vi "Power_spectrum_Autocorrelation.vi"(5 "Spectrum input array":dbl[](array[numeric]) format="%.2f", 7 "Time Trace":T2, 8 "Cluster in":T3={"Colour"=0, "Inst type"=enum."Pitot-static tube", "Inst name"="Manometer voltage", "Symbol"="U", "Code name"="", "Extra Info"="U", "Inst Array"=enum."PWA", "Extra Titles"=[], "Extra Values"=[], "U"=0.0, "u^2"=0.0, "u^3"=0.0, "u^4"=0.0, "Skew_u"=0.0, "Kurt_u"=0.0, "Sd Error in Mean"=0.0, "% u'/U"=0.0, "X"=0.0, "Y"=0.0, "Z"=0.0, "Timescale integral Estimate"=0.0, "Sd Error in Variance"=0.0, "Calib File"=path "", "Calib Constants"=[], "Output Position"=FALSE, "Full Stats"=FALSE, "Av Sampling Rate"=0.0, "Av No of Samples"=0.0, "Total Meas Time (s)"=0.0, "ADAM Ch Name"="", "Max value"=0.0, "Min value"=0.0} {"Sd Error in Variance" format="%.2f"; "Skew_u" format="%.2f"; "% u'/U" format="%.2f"; "Sd Error in Mean" format="%.2f"; "Kurt_u" format="%.2f"; "u^4" format="%.2f"; "u^3" format="%.2f"; "U" format="%.2f"; "u^2" format="%.2f"}) -> (0 "Spectrum output array":dbl[](array[numeric]) format="%.2f", 1 "Autocorrelation":T1, 2 "Spectra":T1, 3 "Cluster Out":T3={"Colour"=0, "Inst type"=enum."Pitot-static tube", "Inst name"="Manometer voltage", "Symbol"="U", "Code name"="", "Extra Info"="U", "Inst Array"=enum."PWA", "Extra Titles"=[], "Extra Values"=[], "U"=0.0, "u^2"=0.0, "u^3"=0.0, "u^4"=0.0, "Skew_u"=0.0, "Kurt_u"=0.0, "Sd Error in Mean"=0.0, "% u'/U"=0.0, "X"=0.0, "Y"=0.0, "Z"=0.0, "Timescale integral Estimate"=0.0, "Sd Error in Variance"=0.0, "Calib File"=path "", "Calib Constants"=[], "Output Position"=FALSE, "Full Stats"=FALSE, "Av Sampling Rate"=0.0, "Av No of Samples"=0.0, "Total Meas Time (s)"=0.0, "ADAM Ch Name"="", "Max value"=0.0, "Min value"=0.0} {"Sd Error in Variance" format="%.2f"; "Skew_u" format="%.2f"; "% u'/U" format="%.2f"; "Sd Error in Mean" format="%.2f"; "Kurt_u" format="%.2f"; "u^4" format="%.2f"; "u^3" format="%.2f"; "U" format="%.2f"; "u^2" format="%.2f"})   [LabVIEW 2016]
uses:
  Controls/Analysis_info_cluster.ctl
  Controls/Inst_type.ctl
  Controls/Instrument_Array.ctl
  Controls/Time_Trace_Cluster.ctl
  Controls/XY_Plot_Cluster.ctl
  Globals/Meas_global.vi
  <vilib>/gmath/NI_Gmath.lvlib
panel:
  out "Numeric":dbl
  out "size(s)":i32
  out "XY Graph 2":cluster{dbl[], dbl[]}(graph)
  in  "method":i32(ring) items=["nearest", "linear", "spline", "cubic Hermite", "Lagrange"]
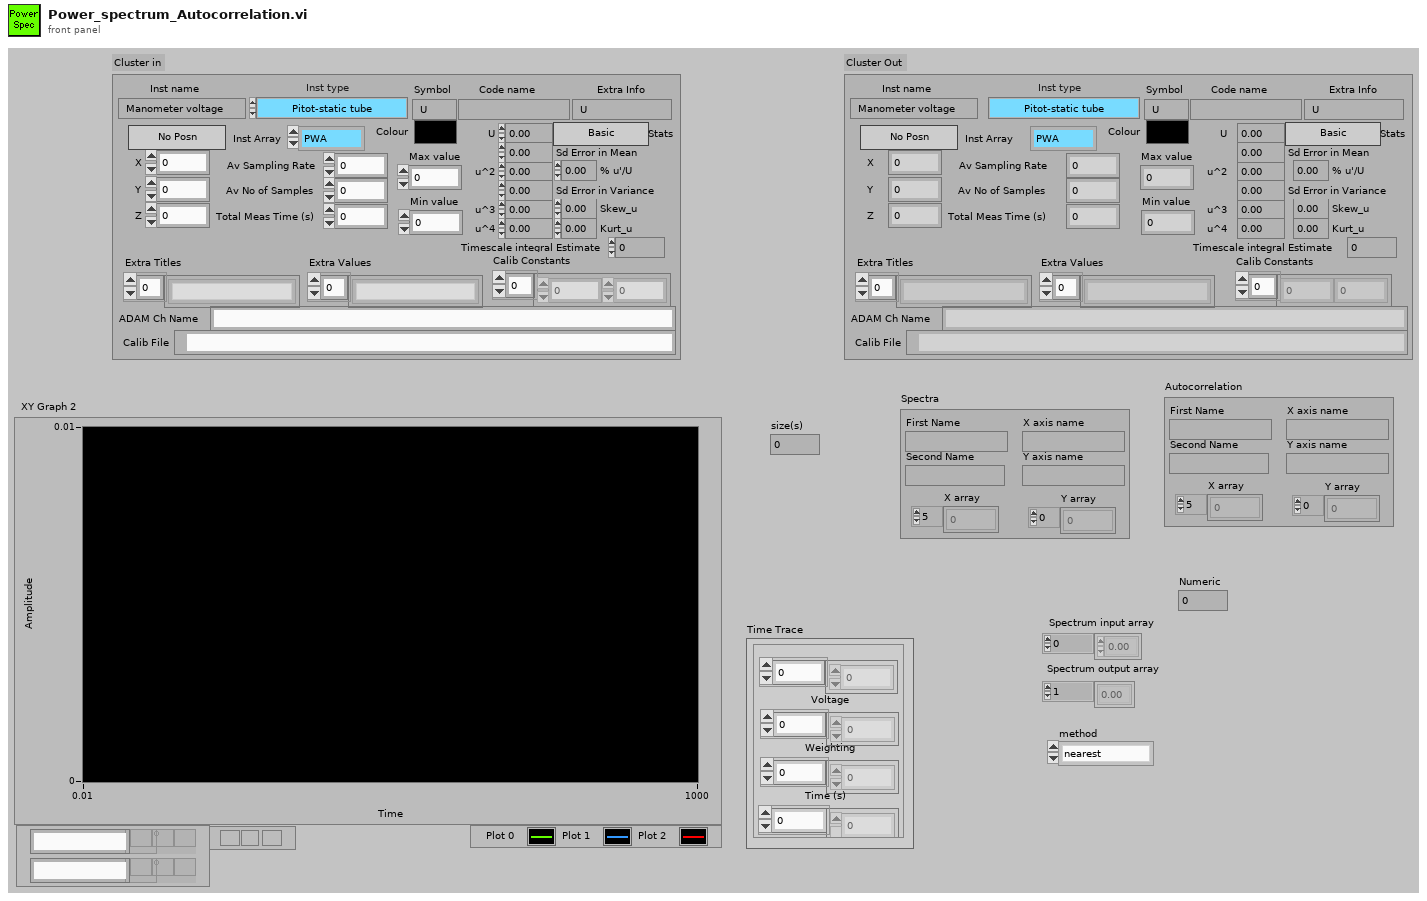
[diagram p1: front panel]
types:
  T1 = typedef "XY_Plot_Cluster.ctl" = cluster{"First Name":string, "Second Name":string, "X axis name":string, "Y axis name":string, "X array":dbl[], "Y array":dbl[]}
  T2 = typedef "Time_Trace_Cluster.ctl" = cluster{"Weighting":dbl[], "Time (s)":dbl[], "Voltage":dbl[], "Eng Values":dbl[]}
  T3 = typedef "Analysis_info_cluster.ctl" = cluster{"Colour":u32, "Inst type":T4, "Inst name":string, "Symbol":string, "Code name":string, "Extra Info":string, "Inst Array":T5, "Extra Titles":string[], "Extra Values":string[], "U":dbl, "u^2":dbl, "u^3":dbl, "u^4":dbl, "Skew_u":dbl, "Kurt_u":dbl, "Sd Error in Mean":dbl, "% u'/U":dbl, "X":dbl, "Y":dbl, "Z":dbl, "Timescale integral Estimate":dbl, "Sd Error in Variance":dbl, "Calib File":path, "Calib Constants":dbl[], "Output Position":bool, "Full Stats":bool, "Av Sampling Rate":dbl, "Av No of Samples":dbl, "Total Meas Time (s)":dbl, "ADAM Ch Name":string, "Max value":dbl, "Min value":dbl}
  T4 = typedef "Inst_type.ctl" = enum16{"Propeller anemometer", "Raw voltage", "Pressure Transducer", "Pitot-static tube", "Preston tube", "Hot wire", "Cross wire 1", "Cross wire 2", "Generic Linear", "Generic Polynomial", "Generic BackPoly", "Fast FID", "Thermocouple", "Cold wire", "Pulsed Wire", "LDA Vel", "LDA Tran time", "LDA Arr time", "Microphone"}
  T5 = typedef "Instrument_Array.ctl" = enum16{"PWA", "LDA", "Analogue"}
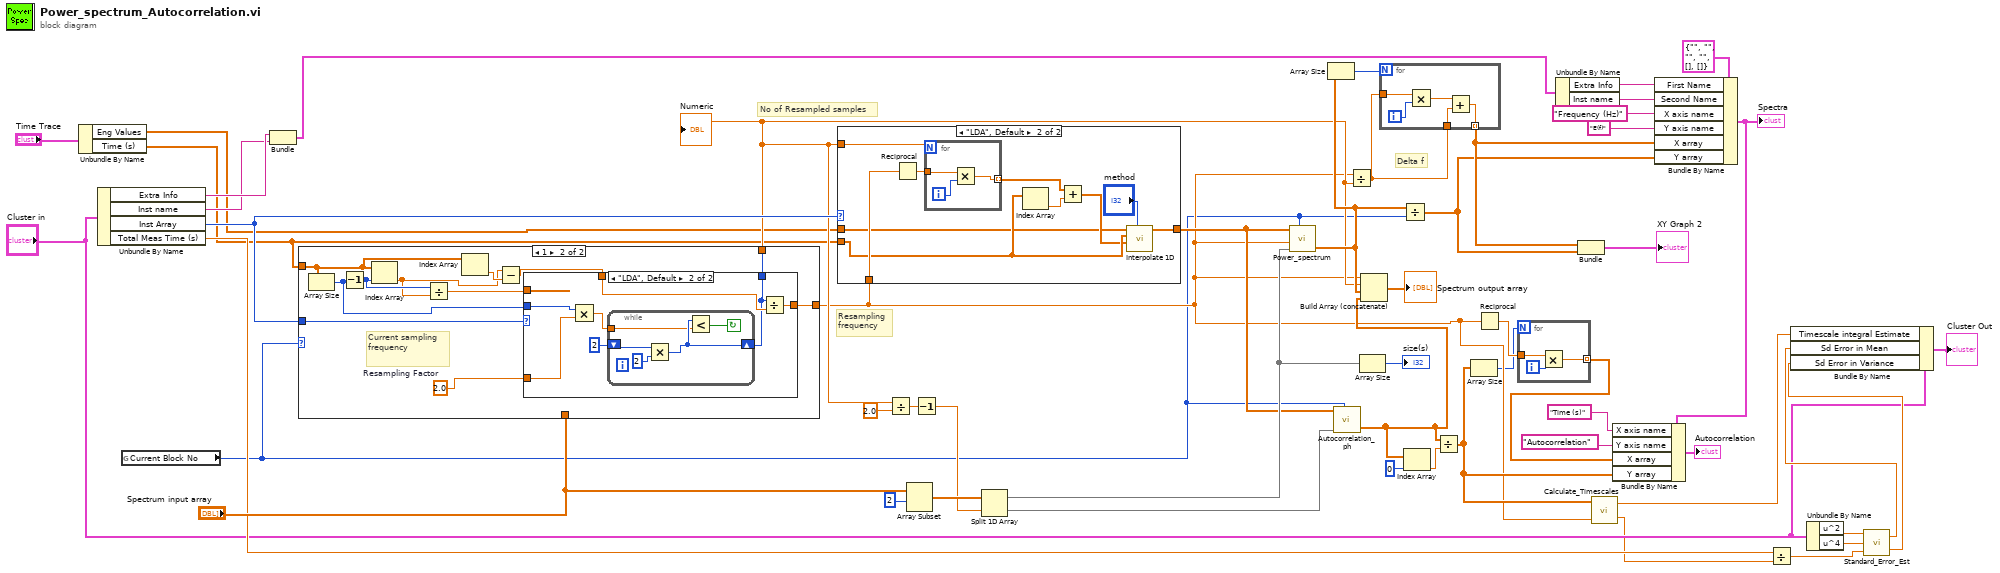
[diagram p0: block diagram]
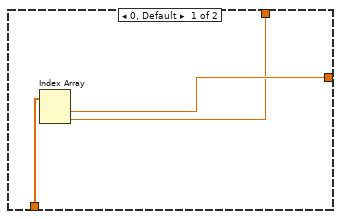
[diagram p2: hidden frame]
diagram:
  # "No of Resampled samples"
  # "Resampling\nfrequency"
  # "Delta f"
  n1 = Unbundle By Name("Time Trace") -> ("Eng Values"=w9:dbl[], "Time (s)"=w5:dbl[])
  n2 = Unbundle By Name("Cluster in") -> ("Extra Info"=w47:string, "Inst name"=w45:string, "Inst Array"=w51:T5, "Total Meas Time (s)"=w11:dbl)
  n3 = global read "Meas_global.vi" "Current Block No"() -> (w3:i32)
  n4 = Bundle("Extra Info"=w47, "Inst name"=w45) -> (w46:cluster{"Extra Info":string, "Inst name":string})  [unwired: 1 in]
  n5 = case shown="1" w3 {
    tunnel: w5 -> [_ w60]
    tunnel: [w55 w65] -> w18
    tunnel: "Spectrum input array" -> [w56 _]
    tunnel: w51 -> [_ w66]
    tunnel: [w54 w63] -> w34
    frame 0, Default {
      n6 = Index Array(array=w56) -> (element #1=w55:dbl, element #2=w54:dbl)  [unwired: 2 in]
    }
    frame 1 {
      w61 = 2.0  # Resampling Factor
      # "Current sampling\nfrequency"
      n7 = Array Size(array=w60) -> (size(s)=w62:i32)
      n8 = Decrement(x=w62) -> (x-1=w64:i32)
      n9 = Index Array(array=w60, index=w64) -> (element=w57:dbl)
      n10 = Divide(x=w64, y=w57) -> (x/y=w67:dbl)
      n11 = Index Array(array=w60) -> (element=w59:dbl)  [unwired: 1 in]
      n12 = Subtract(x=w57, y=w59) -> (x-y=w58:dbl)
      n13 = case shown="\"LDA\", Default" w66 {
        tunnel: w67 -> [w69 _]
        tunnel: w58 -> [_ w76]
        tunnel: [w69 w75] -> w65
        tunnel: w62 -> [w68 w73]
        tunnel: [w68 w72] -> w63
        tunnel: w61 -> [_ w71]
        frame "Analogue" {
        }
        frame "LDA", Default {
          n14 = Multiply(x=w73, y=w71) -> (x*y=w74:dbl)
          n15 = while {
            shift-right: [w79] -> w72
            shift-left: 2 -> [w81]
            tunnel: w74 -> [w77]
            stop <- w78 continue-if-true
            n16 = Multiply(x=w81, y=2) -> (x*y=w79:i32)
            n17 = Less?(x=w79, y=w77) -> (x < y?=w78:bool)
          }
          n18 = Divide(x=w72, y=w76) -> (x/y=w75:dbl)
        }
      }
    }
  }
  "Numeric" <- w34
  n19 = case shown="\"LDA\", Default" w51 {
    tunnel: w9 -> [w82 w83]
    tunnel: w5 -> [_ w87]
    tunnel: [w82 w91] -> w29
    tunnel: w34 -> [_ w90]
    tunnel: w18 -> [_ w88]
    frame "Analogue" {
    }
    frame "LDA", Default {
      n20 = Reciprocal(x=w88) -> (1/x=w89:dbl)
      n21 = for {
        N: w90 -> [_]
        tunnel: w89 -> [w95]
        tunnel: [w93] -> w85 mode=indexing
        i -> [w94]
        n22 = Multiply(x=w95, y=w94) -> (x*y=w93:dbl)
      }
      n23 = Index Array(array=w87) -> (element=w86:dbl)  [unwired: 1 in]
      n24 = Add(x=w85, y=w86) -> (x+y=w84:dbl[])
      n25 = call <vilib>:"Interpolate 1D.vi"("method"="method", "xi"=w84, "X"=w87, "Y"=w83) -> ("yi"=w91:dbl[])  [unwired: 2 in, 5 out]
    }
  }
  n26 = Divide(x=w34, y=2.0) -> (x/y=w32:dbl)
  n27 = Array Subset(array="Spectrum input array", index=2) -> (w35:dbl[])  [unwired: 1 in]
  n28 = Decrement(x=w32) -> (x-1=w31:dbl)
  n29 = Split 1D Array(array=w35, index=w31) -> (first subarray=w30:dbl[], second subarray=w28:dbl[])
  n30 = call "Power_spectrum.vi"("U"=w29, "Sampling frequency"=w18, "Spectrum input array"=w30, "Block No"=w3) -> ("Spectrum Accumulator array"=w39:dbl[])  [unwired: 1 in, 2 out]
  n31 = Array Size(array=w39) -> (size(s)=w49:i32)
  n32 = call "Autocorrelation_ph.vi"("X"=w29, "Autocorrelation of X"=w28, "Block No"=w3) -> ("Autocorrelation of X"=w25:dbl[])  [unwired: 2 in, 1 out]
  n33 = Divide(x=w18, y=w34) -> (x/y=w50:dbl)
  n34 = Array Size(array=w30) -> (size(s)=→"size(s)":i32)
  n35 = Build Array (concatenate)(w18, w34, w39, w25) -> (→"Spectrum output array":dbl[])
  n36 = for {
    N: w49 -> [_]
    tunnel: w50 -> [w100]
    tunnel: w50 -> [w97]
    tunnel: [w96] -> w40 mode=indexing
    i -> [w99]
    n37 = Multiply(x=w100, y=w99) -> (x*y=w98:dbl)
    n38 = Add(x=w98, y=w97) -> (x+y=w96:dbl)
  }
  n39 = Divide(x=w39, y=w3) -> (x/y=w38:dbl[])
  n40 = Index Array(array=w25, index=0 ("Index")) -> (element=w26:dbl)
  n41 = Divide(x=w25, y=w26) -> (x/y=w20:dbl[])
  n42 = Array Size(array=w20) -> (size(s)=w17:i32)
  n43 = Reciprocal(x=w18) -> (1/x=w22:dbl)
  n44 = for {
    N: w17 -> [_]
    tunnel: w22 -> [w102]
    tunnel: [w101] -> w21 mode=indexing
    i -> [w103]
    n45 = Multiply(x=w102, y=w103) -> (x*y=w101:dbl)
  }
  n46 = Unbundle By Name(w46) -> ("Extra Info"=w44:string, "Inst name"=w43:string)
  n47 = Bundle(w40, w38) -> (→"XY Graph 2":cluster{dbl[], dbl[]})  [unwired: 1 in]
  n48 = call "Calculate_Timescales.vi"("Sampling Frequency (Hz)"=w18, "Autocorrelation"=w20) -> ("Time between Independant samples"=w1:dbl, "Timescale estimate (s)"=w2:dbl)  [unwired: 1 in]
  n49 = Bundle By Name(cluster=T1 {"First Name"="", "Second Name"="", "X axis name"="", "Y axis name"="", "X array"=[], "Y array"=[]} ("element"), "First Name"=w44, "Second Name"=w43, "X axis name"="Frequency (Hz)", "Y axis name"="E(f)", "X array"=w40, "Y array"=w38) -> (w7:T1)
  "Spectra" <- w7
  n50 = Bundle By Name(cluster=w7, "X axis name"="Time (s)", "Y axis name"="Autocorrelation", "X array"=w21, "Y array"=w20) -> (→"Autocorrelation":T1)
  n51 = Divide(x=w11, y=w1) -> (x/y=w14:dbl)
  n52 = Unbundle By Name("Cluster in") -> ("u^2"=w16:dbl, "u^4"=w15:dbl)
  n53 = call "Standard_Error_Est.vi"("N"=w14, "4th order moment u^4"=w15, "2nd order moment u^2"=w16) -> ("Standard error in variance"=w12:dbl, "Standard error in Mean"=w13:dbl)
  n54 = Bundle By Name(cluster="Cluster in", "Timescale integral Estimate"=w2, "Sd Error in Mean"=w13, "Sd Error in Variance"=w12) -> (→"Cluster Out":T3)
